vi "Facade.vi"(0 "Data In":T1={25.0, 0.0, 0.0}, 2 "Display State In":T3={"SP_Source"={"connect"=FALSE, "SP_Source"=enum."initialize", "SP_Set"=0.0, "SP"=0.0}, "Write"=FALSE, "button state"=enum."init", "reset_timer"=FALSE, "load_timer"=FALSE, "end_timer"=TRUE}, 3 "Container State":T6) -> (6 "Data Out":T1={25.0, 0.0, 0.0}, 7 "Display State Out":T3={"SP_Source"={"connect"=FALSE, "SP_Source"=enum."initialize", "SP_Set"=0.0, "SP"=0.0}, "Write"=FALSE, "button state"=enum."init", "reset_timer"=FALSE, "load_timer"=FALSE, "end_timer"=TRUE}, 8 "Action":T2)   [LabVIEW 2019, in "Heating.lvlib" / "Y_SP.xctl"]
uses:
  Y_SP.xctl
  Data.ctl
  <vilib>/_xctls/Container State.ctl
  State.ctl
  Z_source.ctl
  Y_controlState.ctl
  <vilib>/_xctls/Action.ctl
  <vilib>/_xctls/XControlSupport.lvlib
  Timer Delay/Timers.lvlib
  Heating.lvlib
panel:
  in  "setpoint":T1={350.0, 0.0, 0.0} caption="oC" scale=0.0..500.0 scale format="%#.1f"
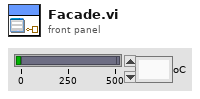
[diagram p1: front panel]
types:
  T1 = typedef "Heating.lvlib/Y_SP.xctl/Data.ctl" = cluster{dbl, dbl, dbl}
  T2 = typedef "XControlSupport.lvlib/Action.ctl" = cluster{"Data Changed?":bool, "State Changed?":bool, "Action Name":string}
  T3 = typedef "Heating.lvlib/Y_SP.xctl/State.ctl" = cluster{"SP_Source":cluster{"connect":bool, "SP_Source":T4, "SP_Set":dbl, "SP":dbl}, "Write":bool, "button state":T5, "reset_timer":bool, "load_timer":bool, "end_timer":bool}
  T4 = typedef "Heating.lvlib/Z_source.ctl" = enum8{"initialize", "local disabled", "local hand", "hand", "auto", "dist"}
  T5 = typedef "Heating.lvlib/Y_SP.xctl/Y_controlState.ctl" = enum16{"init", "not connect", "local disabled", "local hand", "hand", "value change", "auto", "dist"}
  T6 = typedef "XControlSupport.lvlib/Container State.ctl" = cluster{"Indicator?":bool, "Run Mode?":bool, " Refnum":refnum<vi>}
  T7 = enum8{"Enabled", "Disabled", "Disabled and Grayed Out"}
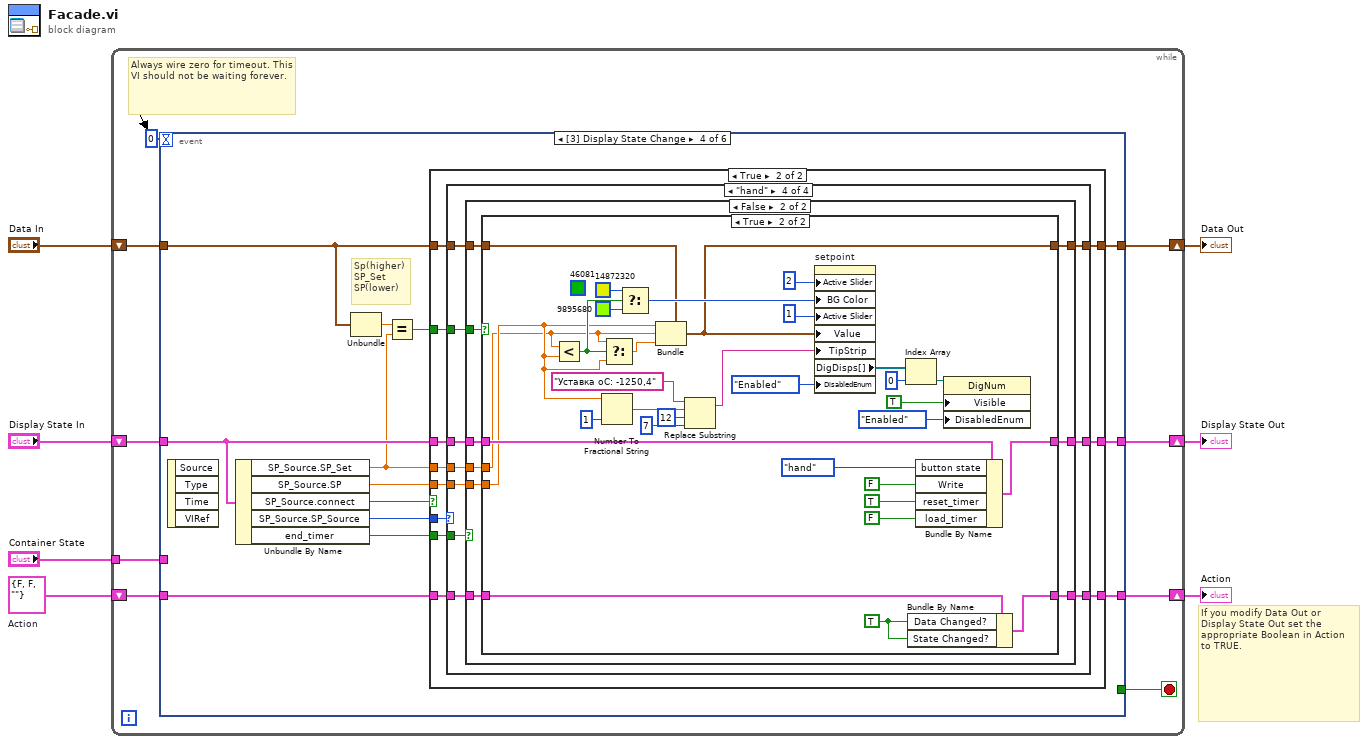
[diagram p0: block diagram]
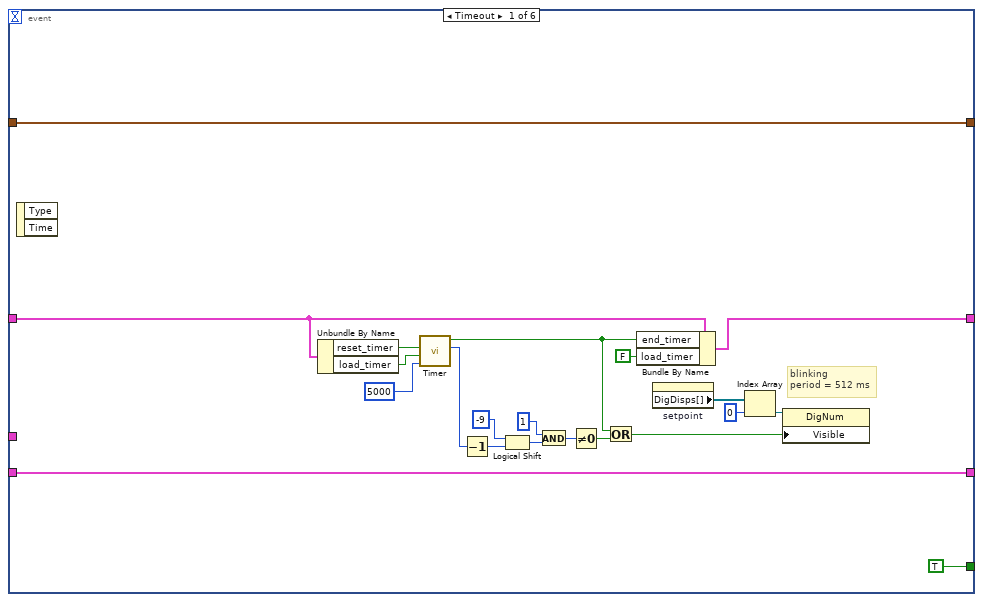
[diagram p2: hidden frame]
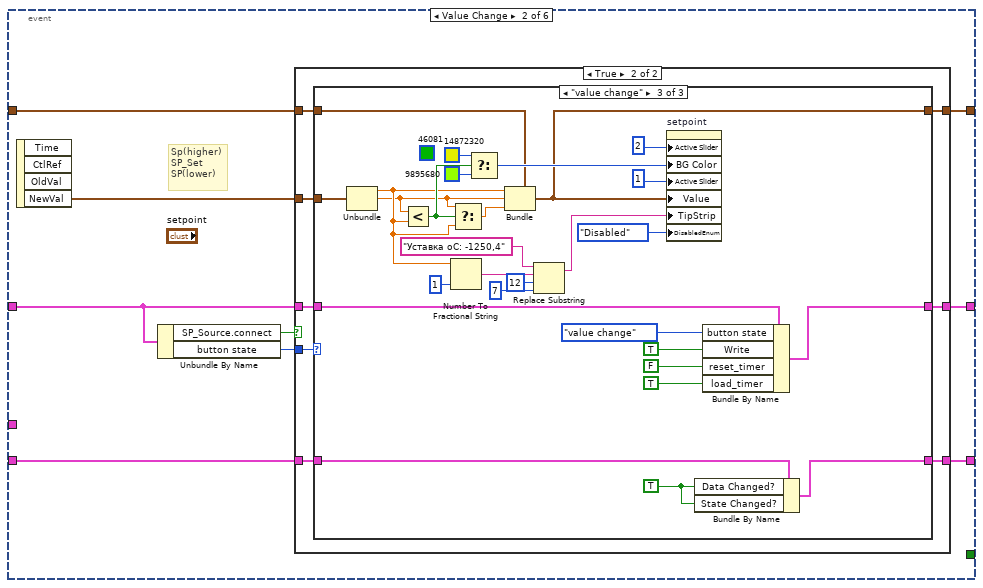
[diagram p3: hidden frame]
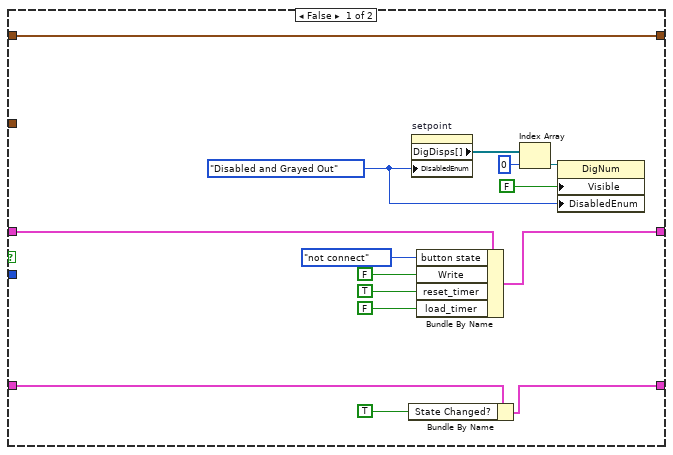
[diagram p4: hidden frame]
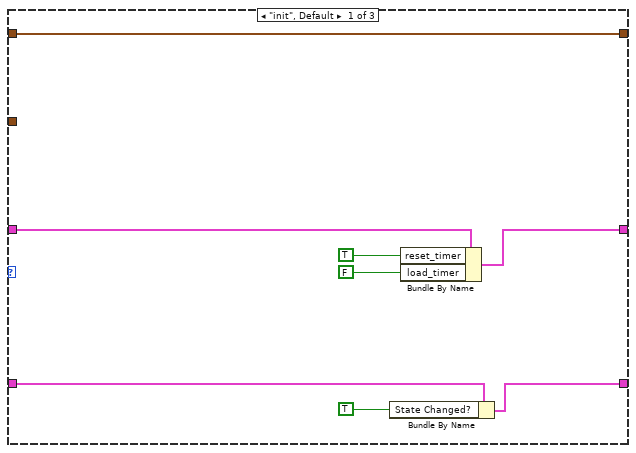
[diagram p5: hidden frame]
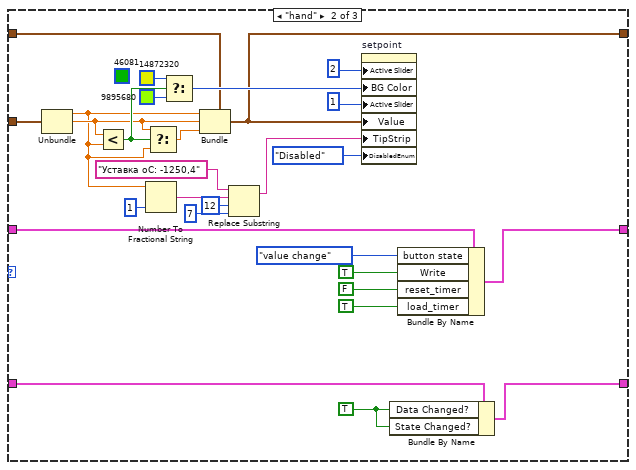
[diagram p6: hidden frame]
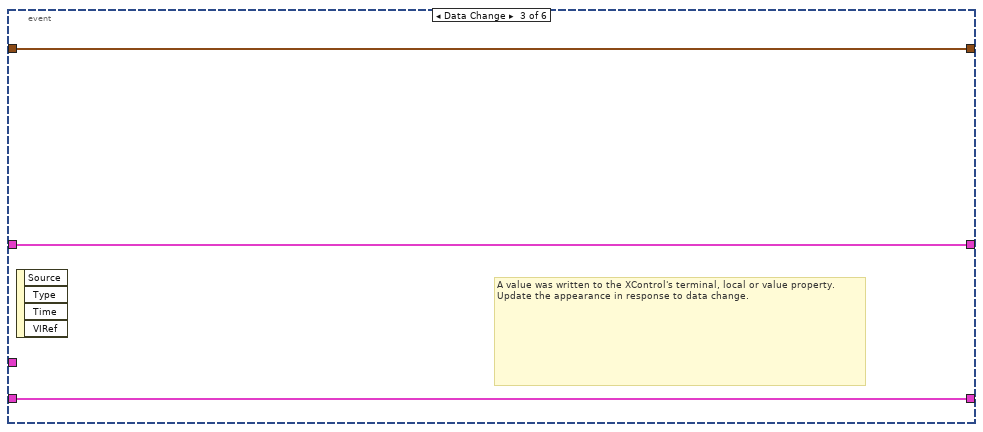
[diagram p7: hidden frame]
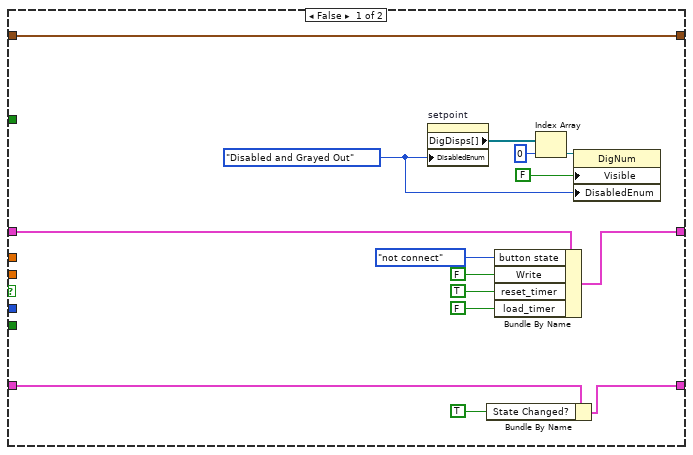
[diagram p8: hidden frame]
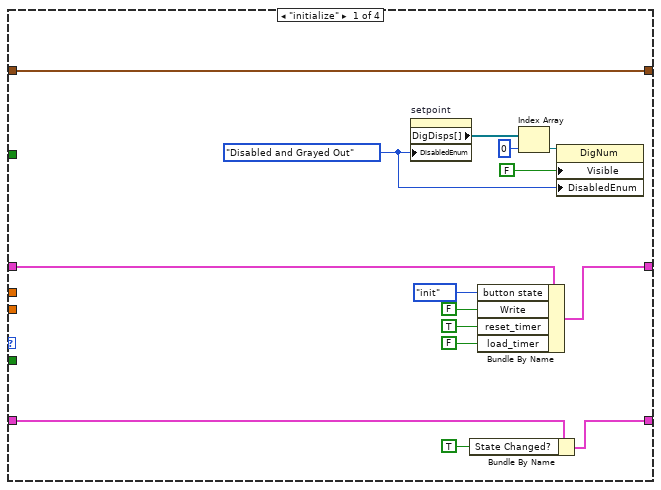
[diagram p9: hidden frame]
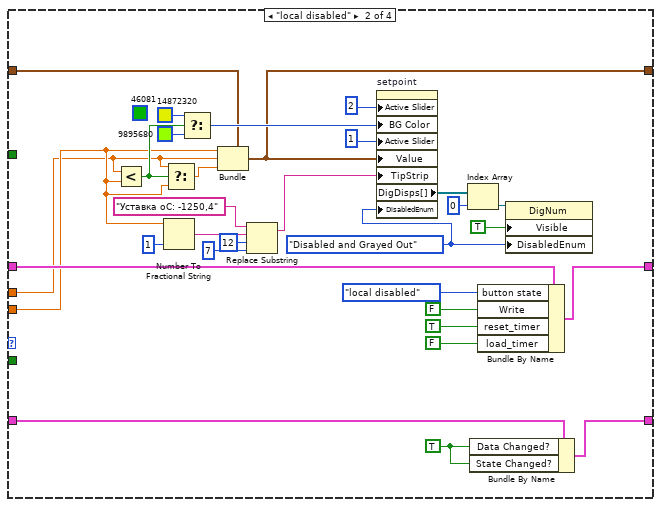
[diagram p10: hidden frame]
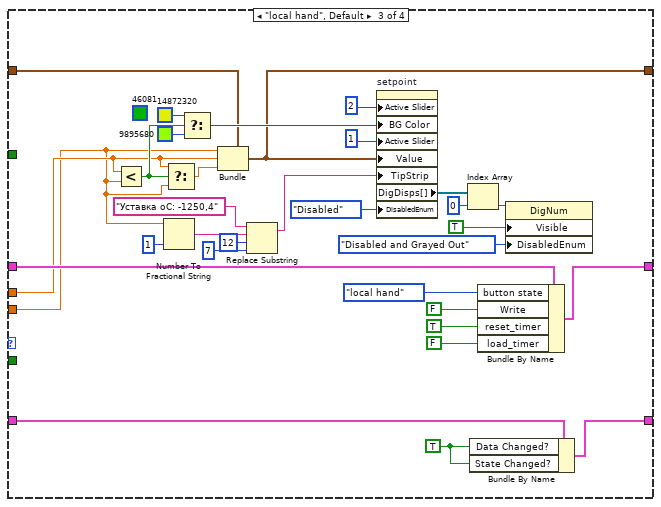
[diagram p11: hidden frame]
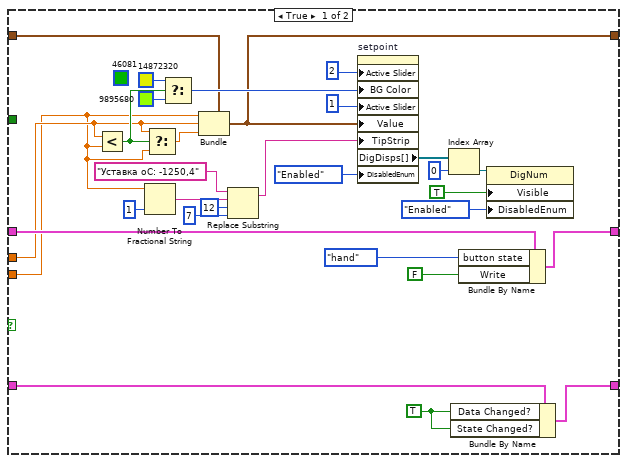
[diagram p12: hidden frame]
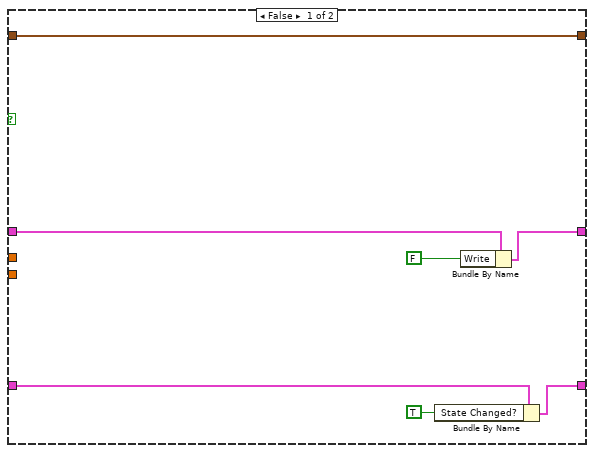
[diagram p13: hidden frame]
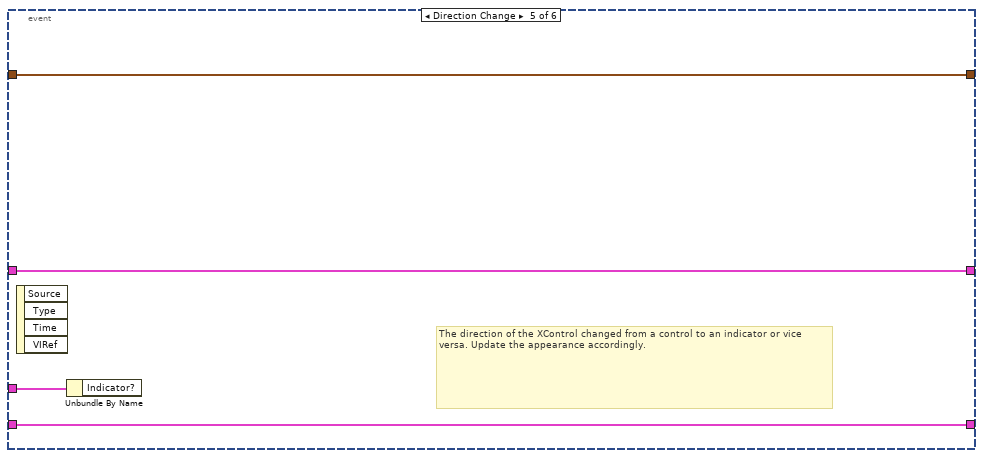
[diagram p14: hidden frame]
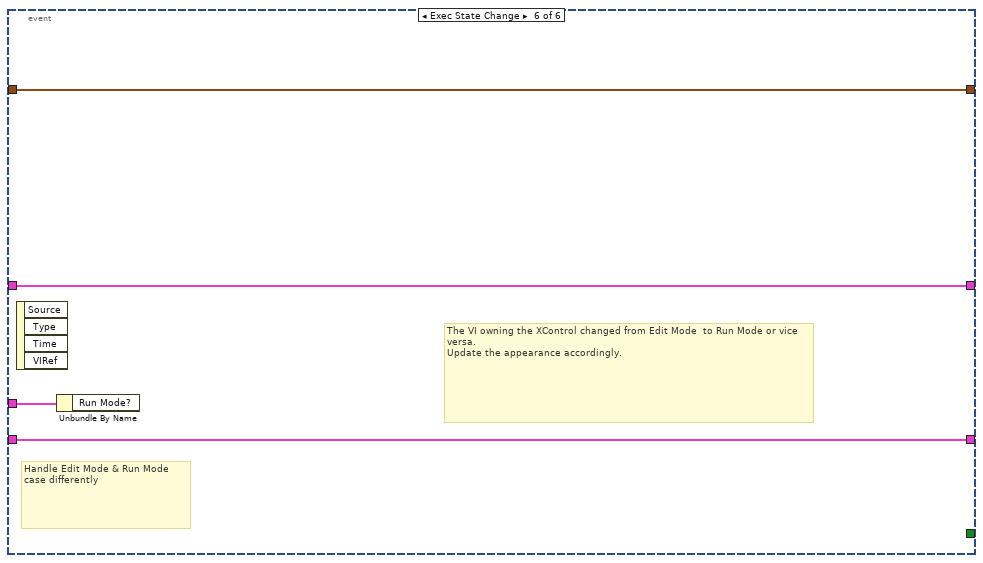
[diagram p15: hidden frame]
diagram:
  w1 = T2 {"Data Changed?"=FALSE, "State Changed?"=FALSE, "Action Name"=""}  # Action
  # "If you modify Data Out or\nDisplay State Out set the\nappropriate Boolean in Action\nto TRUE."
  n1 = while {
    shift-right: [w9] -> w4
    shift-left: "Display State In" -> [w16]
    tunnel: "Container State" -> [w13]
    shift-right: [w8] -> w7
    shift-left: "Data In" -> [w12]
    shift-right: [w10] -> w2
    shift-left: w1 -> [w11]
    stop <- w15 stop-if-true
    # "Always wire zero for timeout. This\nVI should not be waiting forever."
    n2 = event shown="[3] Display State Change" {
      selector: _ -> [_ _ _ _ _ _]
      dyn-events: _ -> [_ _ _ _ _ _]
      timeout: 0 -> [_ _ _ _ _ _]
      tunnel: w16 -> [w32 w41 w135 w144 w344 w348]
      tunnel: [w31 w46 w135 w148 w344 w348] -> w9
      tunnel: [TRUE _ _ _ _ _] -> w15
      tunnel: w13 -> [_ _ _ _ w345 w349]
      tunnel: w12 -> [w35 w45 w136 w139 w343 w347]
      tunnel: [w35 w44 w136 w149 w343 w347] -> w8
      tunnel: [w36 w42 w134 w146 w342 w346] -> w10
      tunnel: w11 -> [w36 w43 w134 w147 w342 w346]
      event Timeout {
        # "blinking\nperiod = 512 ms"
        n3 = event-data() -> ()  [unwired: 1 in, 2 out]
        n4 = Unbundle By Name(w32) -> ("reset_timer"=w34:bool, "load_timer"=w33:bool)
        n5 = call "Timer.vi"("ms"=5000, "Load (F)"=w33, "Reset (F)"=w34) -> ("t ms"=w29:u32, "End"=w26:bool)  [unwired: 6 in]
        n6 = Decrement(x=w29) -> (x-1=w25:u32)
        n7 = Logical Shift(y=i16 -9, x=w25) -> (x << y=w23:u32)
        n8 = And(x=u32 1 ("y"), y=w23) -> (x .and. y?=w21:u32)
        n9 = Not Equal To 0?(x=w21) -> (x != 0?=w27:bool)
        n10 = Or(x=w26, y=w27) -> (x .or. y?=w18:bool)
        n11 = Bundle By Name(cluster=w32, "end_timer"=w26, "load_timer"=FALSE) -> (w31:T3)
        n12 = property on="setpoint" class="Slide (strict)"() -> ("DigDisps[]"=w17:refnum<vi>[])  [unwired: 2 in, 2 out]
        n13 = Index Array(array=w17, index=0) -> (element=w20:refnum<vi>)
        n14 = property class="DigNum"(reference=w20, "Visible"=w18) -> ()  [unwired: 1 in, 2 out]
      }
      event Value Change {
        # "Sp(higher)\nSP_Set\nSP(lower)"
        n15 = event-data() -> ("NewVal"=w38:T1)  [unwired: 1 in, 3 out]
        n16 = Unbundle By Name(w41) -> ("SP_Source.connect"=w40:bool, "button state"=w39:T5)
        n17 = case shown="True" w40 {
          tunnel: w39 -> [_ w69]
          tunnel: w41 -> [w60 w68]
          tunnel: [w59 w67] -> w46
          tunnel: w45 -> [w52 w66]
          tunnel: [w52 w65] -> w44
          tunnel: w43 -> [w57 w63]
          tunnel: [w56 w64] -> w42
          tunnel: w38 -> [_ w62]
          frame False {
            w48 = T7."Disabled and Grayed Out" ("Disabled")
            n18 = Bundle By Name(cluster=w57, "State Changed?"=TRUE ("Data Changed?")) -> (w56:T2)
            n19 = property on="setpoint" class="Slide (strict)"("DisabledEnum"=w48) -> ("DigDisps[]"=w47:refnum<vi>[])  [unwired: 2 in, 2 out]
            n20 = Bundle By Name(cluster=w60, "button state"=Y_controlState."not connect" ("f 3"), "Write"=FALSE ("Z_ASwitch"), "reset_timer"=TRUE ("Z_ASwitch"), "load_timer"=FALSE ("Z_ASwitch")) -> (w59:T3)
            n21 = Index Array(array=w47, index=0) -> (element=w51:refnum<vi>)
            n22 = property class="DigNum"(reference=w51, "Visible"=FALSE ("Z_ASwitch"), "DisabledEnum"=w48) -> ()  [unwired: 1 in, 2 out]
          }
          frame True {
            n23 = case shown="\"value change\"" w69 {
              tunnel: w68 -> [w76 w105 w133]
              tunnel: [w75 w104 w132] -> w67
              tunnel: w66 -> [w70 w82 w110]
              tunnel: [w70 w81 w109] -> w65
              tunnel: [w72 w102 w130] -> w64
              tunnel: w63 -> [w73 w103 w131]
              tunnel: w62 -> [_ w80 w108]
              frame "init", Default {
                # "local hand"
                n24 = Bundle By Name(cluster=w73, "State Changed?"=TRUE ("Data Changed?")) -> (w72:T2)
                n25 = Bundle By Name(cluster=w76, "reset_timer"=TRUE, "load_timer"=FALSE) -> (w75:T3)
              }
              frame "hand" {
                (unwired) u32 46081
                w98 = TRUE ("Data Changed?")
                # "local hand"
                n26 = Unbundle(w80) -> (w78:dbl, w79:dbl)  [unwired: 1 out]
                n27 = Less?(x=w79, y=w78) -> (x < y?=w88:bool)
                n28 = Number To Fractional String(number=w78, precision (6)=i16 1) -> (F-format string=w93:string)  [unwired: 2 in]
                n29 = Select(t=w79, s=w88, f=w78) -> (s? t:f=w87:dbl)
                n30 = Select(t=u32 14872320, s=w88, f=u32 9895680) -> (s? t:f=w83:u32)
                n31 = Bundle(cluster=w82, w78, w79, w87) -> (w81:T1)
                n32 = Replace Substring(2:7 ("length (len. of substring)"), 3:12 ("offset (0)"), 4:w93, 5:"Уставка оС: -1250,4") -> (1:w86:string)  [unwired: 1 out]
                n33 = property on="setpoint" class="Slide (strict)"("Active Slider"=2, "BG Color"=w83, "Active Slider"=1, "Value"=w81, "TipStrip"=w86, "DisabledEnum"=T7."Disabled" ("Disabled")) -> ()  [unwired: 2 in, 2 out]
                n34 = Bundle By Name(cluster=w103, "Data Changed?"=w98, "State Changed?"=w98) -> (w102:T2)
                n35 = Bundle By Name(cluster=w105, "button state"=Y_controlState."value change" ("f 3"), "Write"=TRUE ("Z_ASwitch"), "reset_timer"=FALSE ("Z_ASwitch"), "load_timer"=TRUE ("Z_ASwitch")) -> (w104:T3)
              }
              frame "value change" {
                (unwired) u32 46081
                w126 = TRUE ("Data Changed?")
                # "local hand"
                n36 = Unbundle(w108) -> (w107:dbl, w106:dbl)  [unwired: 1 out]
                n37 = Less?(x=w106, y=w107) -> (x < y?=w116:bool)
                n38 = Number To Fractional String(number=w107, precision (6)=i16 1) -> (F-format string=w121:string)  [unwired: 2 in]
                n39 = Select(t=w106, s=w116, f=w107) -> (s? t:f=w115:dbl)
                n40 = Select(t=u32 14872320, s=w116, f=u32 9895680) -> (s? t:f=w111:u32)
                n41 = Bundle(cluster=w110, w107, w106, w115) -> (w109:T1)
                n42 = Replace Substring(2:7 ("length (len. of substring)"), 3:12 ("offset (0)"), 4:w121, 5:"Уставка оС: -1250,4") -> (1:w114:string)  [unwired: 1 out]
                n43 = property on="setpoint" class="Slide (strict)"("Active Slider"=2, "BG Color"=w111, "Active Slider"=1, "Value"=w109, "TipStrip"=w114, "DisabledEnum"=T7."Disabled" ("Disabled")) -> ()  [unwired: 2 in, 2 out]
                n44 = Bundle By Name(cluster=w131, "Data Changed?"=w126, "State Changed?"=w126) -> (w130:T2)
                n45 = Bundle By Name(cluster=w133, "button state"=Y_controlState."value change" ("f 3"), "Write"=TRUE ("Z_ASwitch"), "reset_timer"=FALSE ("Z_ASwitch"), "load_timer"=TRUE ("Z_ASwitch")) -> (w132:T3)
              }
            }
          }
        }
      }
      event Data Change {
        # "A value was written to the XControl's terminal, local or value property.\nUpdate the appearance in response to data change."
        n46 = event-data() -> ()  [unwired: 1 in, 4 out]
      }
      event Display State Change {
        # "Sp(higher)\nSP_Set\nSP(lower)"
        n47 = event-data() -> ()  [unwired: 1 in, 4 out]
        n48 = Unbundle By Name(w144) -> ("SP_Source.SP_Set"=w137:dbl, "SP_Source.SP"=w140:dbl, "SP_Source.connect"=w145:bool, "SP_Source.SP_Source"=w142:T4, "end_timer"=w143:bool)
        n49 = Unbundle(w139) -> (w138:dbl)  [unwired: 2 out]
        n50 = Equal?(x=w138, y=w137) -> (x = y?=w141:bool)
        n51 = case shown="True" w145 {
          tunnel: w142 -> [_ w175]
          tunnel: w144 -> [w163 w174]
          tunnel: [w162 w173] -> w148
          tunnel: w139 -> [w151 w172]
          tunnel: [w151 w171] -> w149
          tunnel: w147 -> [w160 w169]
          tunnel: [w159 w170] -> w146
          tunnel: w143 -> [_ w168]
          tunnel: w140 -> [_ w167]
          tunnel: w141 -> [_ w166]
          tunnel: w137 -> [_ w165]
          frame False {
            w150 = T7."Disabled and Grayed Out" ("Disabled")
            n52 = property on="setpoint" class="Slide (strict)"("DisabledEnum"=w150) -> ("DigDisps[]"=w154:refnum<vi>[])  [unwired: 2 in, 2 out]
            n53 = Bundle By Name(cluster=w160, "State Changed?"=TRUE ("Data Changed?")) -> (w159:T2)
            n54 = Bundle By Name(cluster=w163, "button state"=Y_controlState."not connect" ("f 3"), "Write"=FALSE ("Z_ASwitch"), "reset_timer"=TRUE ("Z_ASwitch"), "load_timer"=FALSE ("Z_ASwitch")) -> (w162:T3)
            n55 = Index Array(array=w154, index=0) -> (element=w155:refnum<vi>)
            n56 = property class="DigNum"(reference=w155, "Visible"=FALSE ("Z_ASwitch"), "DisabledEnum"=w150) -> ()  [unwired: 1 in, 2 out]
          }
          frame True {
            n57 = case shown="\"hand\"" w175 {
              tunnel: w174 -> [w190 w221 w253 w263]
              tunnel: [w189 w220 w252 w262] -> w173
              tunnel: w172 -> [w176 w195 w225 w256]
              tunnel: [w176 w194 w224 w257] -> w171
              tunnel: [w187 w218 w250 w260] -> w170
              tunnel: w169 -> [w188 w219 w251 w261]
              tunnel: w168 -> [_ _ _ w259]
              tunnel: w167 -> [_ w193 w222 w258]
              tunnel: w166 -> [_ _ _ w255]
              tunnel: w165 -> [_ w192 w223 w254]
              frame "initialize" {
                w181 = T7."Disabled and Grayed Out" ("Disabled")
                # "local hand"
                n58 = property on="setpoint" class="Slide (strict)"("DisabledEnum"=w181) -> ("DigDisps[]"=w179:refnum<vi>[])  [unwired: 2 in, 2 out]
                n59 = Bundle By Name(cluster=w188, "State Changed?"=TRUE ("Data Changed?")) -> (w187:T2)
                n60 = Bundle By Name(cluster=w190, "button state"=Y_controlState."init" ("f 3"), "Write"=FALSE ("Z_ASwitch"), "reset_timer"=TRUE ("Z_ASwitch"), "load_timer"=FALSE ("Z_ASwitch")) -> (w189:T3)
                n61 = Index Array(array=w179, index=0) -> (element=w180:refnum<vi>)
                n62 = property class="DigNum"(reference=w180, "Visible"=FALSE ("Z_ASwitch"), "DisabledEnum"=w181) -> ()  [unwired: 1 in, 2 out]
              }
              frame "local disabled" {
                (unwired) u32 46081
                w191 = T7."Disabled and Grayed Out" ("Disabled")
                w213 = TRUE ("Data Changed?")
                # "local hand"
                n63 = Less?(x=w192, y=w193) -> (x < y?=w202:bool)
                n64 = Number To Fractional String(number=w193, precision (6)=i16 1) -> (F-format string=w207:string)  [unwired: 2 in]
                n65 = Select(t=w192, s=w202, f=w193) -> (s? t:f=w201:dbl)
                n66 = Select(t=u32 14872320, s=w202, f=u32 9895680) -> (s? t:f=w197:u32)
                n67 = Bundle(cluster=w195, w193, w192, w201) -> (w194:T1)
                n68 = Replace Substring(2:7 ("length (len. of substring)"), 3:12 ("offset (0)"), 4:w207, 5:"Уставка оС: -1250,4") -> (1:w200:string)  [unwired: 1 out]
                n69 = property on="setpoint" class="Slide (strict)"("Active Slider"=2, "BG Color"=w197, "Active Slider"=1, "Value"=w194, "TipStrip"=w200, "DisabledEnum"=w191) -> ("DigDisps[]"=w196:refnum<vi>[])  [unwired: 2 in, 2 out]
                n70 = Index Array(array=w196, index=0) -> (element=w212:refnum<vi>)
                n71 = Bundle By Name(cluster=w219, "Data Changed?"=w213, "State Changed?"=w213) -> (w218:T2)
                n72 = Bundle By Name(cluster=w221, "button state"=Y_controlState."local disabled" ("f 3"), "Write"=FALSE ("Z_ASwitch"), "reset_timer"=TRUE ("Z_ASwitch"), "load_timer"=FALSE ("Z_ASwitch")) -> (w220:T3)
                n73 = property class="DigNum"(reference=w212, "Visible"=TRUE ("Z_ASwitch"), "DisabledEnum"=w191) -> ()  [unwired: 1 in, 2 out]
              }
              frame "local hand", Default {
                (unwired) u32 46081
                w245 = TRUE ("Data Changed?")
                # "local hand"
                n74 = Less?(x=w223, y=w222) -> (x < y?=w232:bool)
                n75 = Number To Fractional String(number=w222, precision (6)=i16 1) -> (F-format string=w237:string)  [unwired: 2 in]
                n76 = Select(t=w223, s=w232, f=w222) -> (s? t:f=w231:dbl)
                n77 = Select(t=u32 14872320, s=w232, f=u32 9895680) -> (s? t:f=w227:u32)
                n78 = Bundle(cluster=w225, w222, w223, w231) -> (w224:T1)
                n79 = Replace Substring(2:7 ("length (len. of substring)"), 3:12 ("offset (0)"), 4:w237, 5:"Уставка оС: -1250,4") -> (1:w230:string)  [unwired: 1 out]
                n80 = property on="setpoint" class="Slide (strict)"("Active Slider"=2, "BG Color"=w227, "Active Slider"=1, "Value"=w224, "TipStrip"=w230, "DisabledEnum"=T7."Disabled" ("Disabled")) -> ("DigDisps[]"=w226:refnum<vi>[])  [unwired: 2 in, 2 out]
                n81 = Index Array(array=w226, index=0) -> (element=w244:refnum<vi>)
                n82 = Bundle By Name(cluster=w251, "Data Changed?"=w245, "State Changed?"=w245) -> (w250:T2)
                n83 = Bundle By Name(cluster=w253, "button state"=Y_controlState."local hand" ("f 3"), "Write"=FALSE ("Z_ASwitch"), "reset_timer"=TRUE ("Z_ASwitch"), "load_timer"=FALSE ("Z_ASwitch")) -> (w252:T3)
                n84 = property class="DigNum"(reference=w244, "Visible"=TRUE ("Z_ASwitch"), "DisabledEnum"=T7."Disabled and Grayed Out" ("Disabled")) -> ()  [unwired: 1 in, 2 out]
              }
              frame "hand" {
                # "local hand"
                n85 = case shown="False" w259 {
                  tunnel: w263 -> [w293 w302]
                  tunnel: [w292 w301] -> w262
                  tunnel: w261 -> [w291 w300]
                  tunnel: [w290 w299] -> w260
                  tunnel: w258 -> [w265 w296]
                  tunnel: [w264 w298] -> w257
                  tunnel: w256 -> [w267 w297]
                  tunnel: w255 -> [_ w295]
                  tunnel: w254 -> [w266 w294]
                  frame True {
                    (unwired) u32 46081
                    w287 = TRUE ("Data Changed?")
                    n86 = Less?(x=w266, y=w265) -> (x < y?=w273:bool)
                    n87 = Number To Fractional String(number=w265, precision (6)=i16 1) -> (F-format string=w278:string)  [unwired: 2 in]
                    n88 = Select(t=w266, s=w273, f=w265) -> (s? t:f=w272:dbl)
                    n89 = Select(t=u32 14872320, s=w273, f=u32 9895680) -> (s? t:f=w268:u32)
                    n90 = Bundle(cluster=w267, w265, w266, w272) -> (w264:T1)
                    n91 = Replace Substring(2:7 ("length (len. of substring)"), 3:12 ("offset (0)"), 4:w278, 5:"Уставка оС: -1250,4") -> (1:w271:string)  [unwired: 1 out]
                    n92 = property on="setpoint" class="Slide (strict)"("Active Slider"=2, "BG Color"=w268, "Active Slider"=1, "Value"=w264, "TipStrip"=w271, "DisabledEnum"=T7."Enabled" ("Disabled")) -> ("DigDisps[]"=w284:refnum<vi>[])  [unwired: 2 in, 2 out]
                    n93 = Index Array(array=w284, index=0) -> (element=w285:refnum<vi>)
                    n94 = Bundle By Name(cluster=w291, "Data Changed?"=w287, "State Changed?"=w287) -> (w290:T2)
                    n95 = Bundle By Name(cluster=w293, "button state"=Y_controlState."hand" ("f 3"), "Write"=FALSE ("Z_ASwitch")) -> (w292:T3)
                    n96 = property class="DigNum"(reference=w285, "Visible"=TRUE ("Z_ASwitch"), "DisabledEnum"=T7."Enabled" ("Disabled")) -> ()  [unwired: 1 in, 2 out]
                  }
                  frame False {
                    n97 = case shown="True" w295 {
                      tunnel: w302 -> [w305 w341]
                      tunnel: [w304 w340] -> w301
                      tunnel: w300 -> [w308 w339]
                      tunnel: [w306 w338] -> w299
                      tunnel: [w309 w311] -> w298
                      tunnel: w297 -> [w309 w310]
                      tunnel: w296 -> [_ w316]
                      tunnel: w294 -> [_ w315]
                      frame False {
                        n98 = Bundle By Name(cluster=w308, "State Changed?"=TRUE ("Data Changed?")) -> (w306:T2)
                        n99 = Bundle By Name(cluster=w305, "Write"=FALSE ("Z_ASwitch")) -> (w304:T3)
                      }
                      frame True {
                        (unwired) u32 46081
                        w335 = TRUE ("Data Changed?")
                        n100 = Less?(x=w315, y=w316) -> (x < y?=w319:bool)
                        n101 = Number To Fractional String(number=w316, precision (6)=i16 1) -> (F-format string=w324:string)  [unwired: 2 in]
                        n102 = Select(t=w315, s=w319, f=w316) -> (s? t:f=w318:dbl)
                        n103 = Select(t=u32 14872320, s=w319, f=u32 9895680) -> (s? t:f=w312:u32)
                        n104 = Bundle(cluster=w310, w316, w315, w318) -> (w311:T1)
                        n105 = Replace Substring(2:7 ("length (len. of substring)"), 3:12 ("offset (0)"), 4:w324, 5:"Уставка оС: -1250,4") -> (1:w317:string)  [unwired: 1 out]
                        n106 = property on="setpoint" class="Slide (strict)"("Active Slider"=2, "BG Color"=w312, "Active Slider"=1, "Value"=w311, "TipStrip"=w317, "DisabledEnum"=T7."Enabled" ("Disabled")) -> ("DigDisps[]"=w332:refnum<vi>[])  [unwired: 2 in, 2 out]
                        n107 = Index Array(array=w332, index=0) -> (element=w333:refnum<vi>)
                        n108 = Bundle By Name(cluster=w339, "Data Changed?"=w335, "State Changed?"=w335) -> (w338:T2)
                        n109 = Bundle By Name(cluster=w341, "button state"=Y_controlState."hand" ("f 3"), "Write"=FALSE ("Z_ASwitch"), "reset_timer"=TRUE ("Z_ASwitch"), "load_timer"=FALSE ("Z_ASwitch")) -> (w340:T3)
                        n110 = property class="DigNum"(reference=w333, "Visible"=TRUE ("Z_ASwitch"), "DisabledEnum"=T7."Enabled" ("Disabled")) -> ()  [unwired: 1 in, 2 out]
                      }
                    }
                  }
                }
              }
            }
          }
        }
      }
      event Direction Change {
        # "The direction of the XControl changed from a control to an indicator or vice versa. Update the appearance accordingly."
        n111 = event-data() -> ()  [unwired: 1 in, 4 out]
        n112 = Unbundle By Name(w345) -> ()  [unwired: 1 out]
      }
      event Exec State Change {
        # "The VI owning the XControl changed from Edit Mode  to Run Mode or vice versa.\nUpdate the appearance accordingly."
        # "Handle Edit Mode & Run Mode\ncase differently"
        n113 = event-data() -> ()  [unwired: 1 in, 4 out]
        n114 = Unbundle By Name(w349) -> ()  [unwired: 1 out]
      }
    }
  }
  "Display State Out" <- w4
  "Data Out" <- w7
  "Action" <- w2
